vi "StopAxis.vi"(4 "error in (no error)":errorcluster, 6 "timeout":u32, 7 "axis in":cluster{"keyHandle":u32, "nodeId":u16}={"keyHandle"=0, "nodeId"=1}) -> (0 "error out":errorcluster, 3 "axis out":cluster{"keyHandle":u32, "nodeId":u16}={"keyHandle"=0, "nodeId"=1})   [LabVIEW 2019]
doc: "<B>StopAxis</B> stops the positioning or the movement. The function is depends on the operational mode."
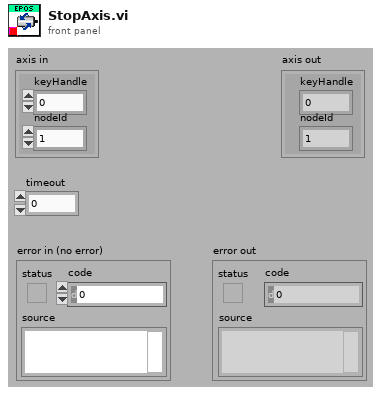
[diagram p1: front panel]
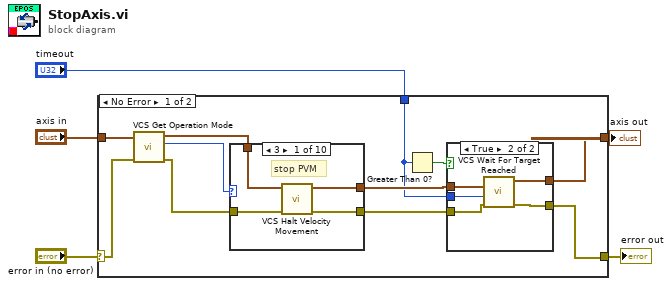
[diagram p0: block diagram]
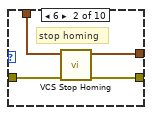
[diagram p3: hidden frame]
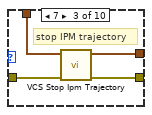
[diagram p4: hidden frame]
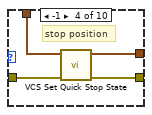
[diagram p5: hidden frame]
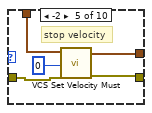
[diagram p6: hidden frame]
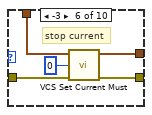
[diagram p7: hidden frame]
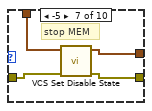
[diagram p8: hidden frame]
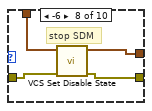
[diagram p9: hidden frame]
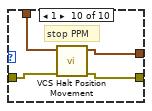
[diagram p11: hidden frame]
diagram:
  n1 = case shown="No Error" "error in (no error)" {
    selector: "error in (no error)" -> [w14 w65]
    tunnel: [w6 w65] -> w4
    tunnel: [w7 w64] -> w3
    tunnel: "axis in" -> [w16 w64]
    tunnel: "timeout" -> [w8 _]
    frame No Error {
      n2 = call "VCS Get Operation Mode.vi"("error in (no error)"=w14, "axis in"=w16) -> ("error out"=w12:errorcluster, "modes of operations"=w15:i8, "axis out"=w13:cluster{"keyHandle":u32, "nodeId":u16})  [unwired: 7 in]
      n3 = case shown="3" w15 {
        tunnel: w13 -> [w24 w31 w35 w36 w44 w46 w50 w54 w59 w60]
        tunnel: [w27 w30 w34 w39 w40 w49 w53 w55 w59 w63] -> w9
        tunnel: [w26 w29 w33 w38 w41 w48 w52 w56 w58 w62] -> w10
        tunnel: w12 -> [w25 w28 w32 w37 w42 w47 w51 w57 w58 w61]
        frame 3 {
          # "stop PVM"
          n4 = call "VCS Halt Velocity Movement.vi"("error in (no error)"=w25, "axis in"=w24) -> ("error out"=w26:errorcluster, "axis out"=w27:cluster{"keyHandle":u32, "nodeId":u16})  [unwired: 8 in]
        }
        frame 6 {
          # "stop homing"
          n5 = call "VCS Stop Homing.vi"("error in (no error)"=w28, "axis in"=w31) -> ("error out"=w29:errorcluster, "axis out"=w30:cluster{"keyHandle":u32, "nodeId":u16})  [unwired: 8 in]
        }
        frame 7 {
          # "stop IPM trajectory"
          n6 = call "VCS Stop Ipm Trajectory.vi"("error in (no error)"=w32, "axis in"=w35) -> ("error out"=w33:errorcluster, "axis out"=w34:cluster{"keyHandle":u32, "nodeId":u16})  [unwired: 8 in]
        }
        frame -1 {
          # "stop position"
          n7 = call "VCS Set Quick Stop State.vi"("error in (no error)"=w37, "axis in"=w36) -> ("error out"=w38:errorcluster, "axis out"=w39:cluster{"keyHandle":u32, "nodeId":u16})  [unwired: 8 in]
        }
        frame -2 {
          # "stop velocity"
          n8 = call "VCS Set Velocity Must.vi"("error in (no error)"=w42, "velocityMust"=0, "axis in"=w44) -> ("error out"=w41:errorcluster, "axis out"=w40:cluster{"keyHandle":u32, "nodeId":u16})  [unwired: 7 in]
        }
        frame -3 {
          # "stop current"
          n9 = call "VCS Set Current Must.vi"("error in (no error)"=w47, "currentMust"=i16 0, "axis in"=w46) -> ("error out"=w48:errorcluster, "axis out"=w49:cluster{"keyHandle":u32, "nodeId":u16})  [unwired: 7 in]
        }
        frame -5 {
          # "stop MEM"
          n10 = call "VCS Set Disable State.vi"("error in (no error)"=w51, "axis in"=w50) -> ("error out"=w52:errorcluster, "axis out"=w53:cluster{"keyHandle":u32, "nodeId":u16})  [unwired: 8 in]
        }
        frame -6 {
          # "stop SDM"
          n11 = call "VCS Set Disable State.vi"("error in (no error)"=w57, "axis in"=w54) -> ("error out"=w56:errorcluster, "axis out"=w55:cluster{"keyHandle":u32, "nodeId":u16})  [unwired: 8 in]
        }
        frame Default {
          # "undefined"
        }
        frame 1 {
          # "stop PPM"
          n12 = call "VCS Halt Position Movement.vi"("error in (no error)"=w61, "axis in"=w60) -> ("error out"=w62:errorcluster, "axis out"=w63:cluster{"keyHandle":u32, "nodeId":u16})  [unwired: 8 in]
        }
      }
      n13 = Greater Than 0?(x=w8) -> (x > 0?=w11:bool)
      n14 = case shown="True" w11 {
        tunnel: [w18 w23] -> w7
        tunnel: [w17 w22] -> w6
        tunnel: w10 -> [w17 w21]
        tunnel: w9 -> [w18 w20]
        tunnel: w8 -> [_ w19]
        frame False {
        }
        frame True {
          n15 = call "VCS Wait For Target Reached.vi"("error in (no error)"=w21, "timeout"=w19, "axis in"=w20) -> ("error out"=w22:errorcluster, "axis out"=w23:cluster{"keyHandle":u32, "nodeId":u16})  [unwired: 7 in]
        }
      }
    }
    frame Error {
    }
  }
  "error out" <- w4
  "axis out" <- w3
